vi "State Machine Fundamentals.vi"() -> ()   [LabVIEW 2014]
doc: "Demonstrates the fundamentals of the State Machine design pattern in LabVIEW. A state machine, in its simplest form, is a case structure within a while loop, with a state enum wired to a shift register on the loop to define the execution of different cases (or \"states\") of the case structure on different iterations of the loop."
uses:
  Program Files (x86)/National Instruments/LabVIEW 2014/examples/Design Patterns/State Machine/support/State Machine Fundamentals - State Enum.ctl
panel:
  in  "No":string="No"
  in  "Yes":string="Yes"
  in  "State 3 Text":string="State 3 is executing."
  in  "State 2 Text":string="State 2 is executing. Do you want to execute State 3 next?"
  in  "State 1 Text":string="State 1 is executing."
  in  "Stop":bool
  in  "Run State 2":bool
  in  "Run State 1":bool
  # "Overview: Demonstrates the fundamental concepts of a State Machine design pattern in LabVIEW.\nInstructions:\n1. Run the VI.\n2. Click the Run State 1 button. A dialog pops up displaying text.\n3. Click the Run State 2 button. If you select \"Yes\" in the pop up dialog, State 3 will run after State 2.\n4. Click Stop to stop the VI."
  # "Note: If you are creating a LabVIEW application based on the state machine design pattern, create a Simple State Machine project from the File > Create Project dialog."
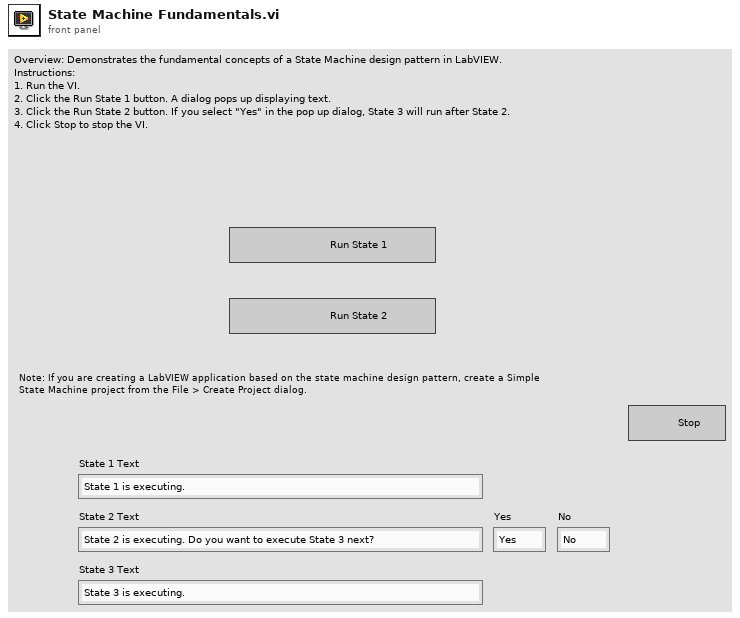
[diagram p1: front panel]
types:
  T1 = typedef "State Machine Fundamentals - State Enum.ctl" = enum16{"Initialize", "Wait for Event", "State 1", "State 2", "State 3", "Stop"}
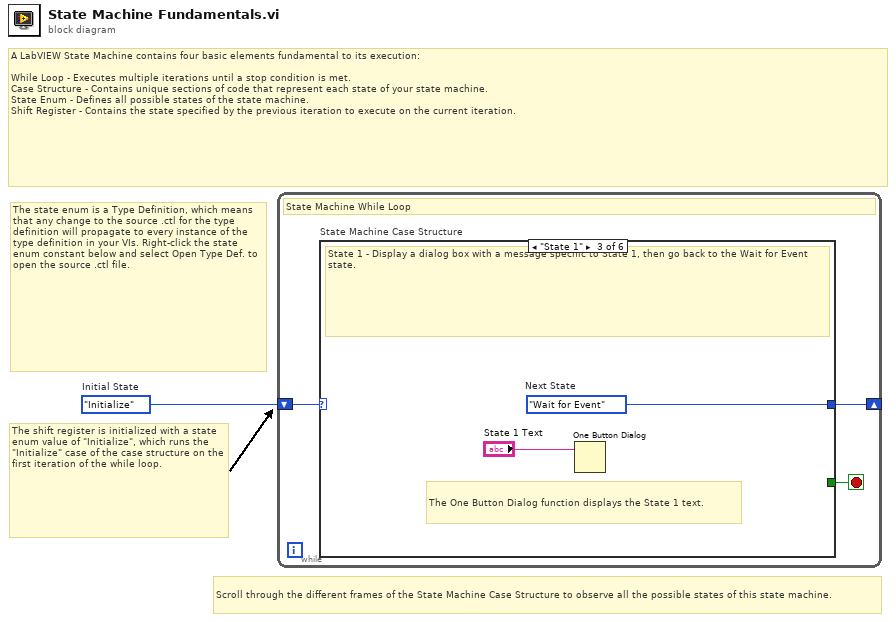
[diagram p0: block diagram]
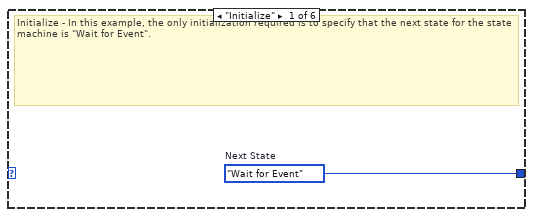
[diagram p2: hidden frame]
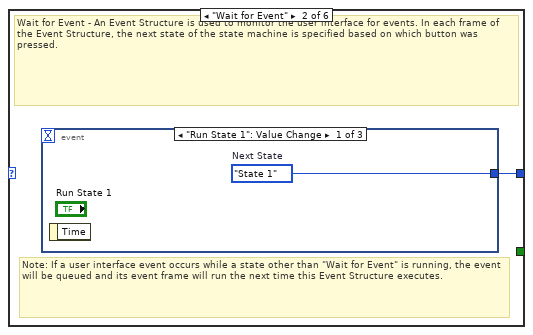
[diagram p3: hidden frame]
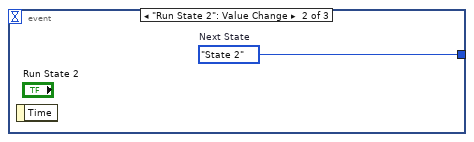
[diagram p4: hidden frame]
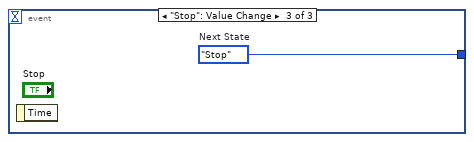
[diagram p5: hidden frame]
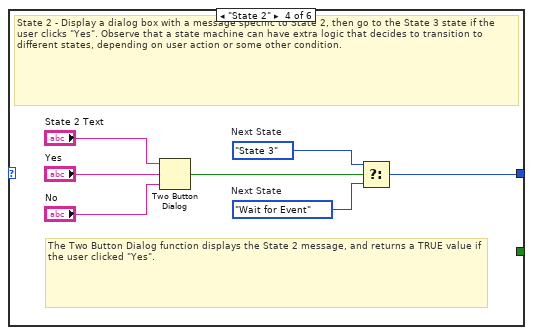
[diagram p6: hidden frame]
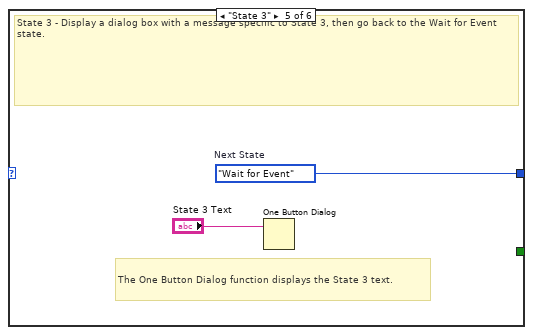
[diagram p7: hidden frame]
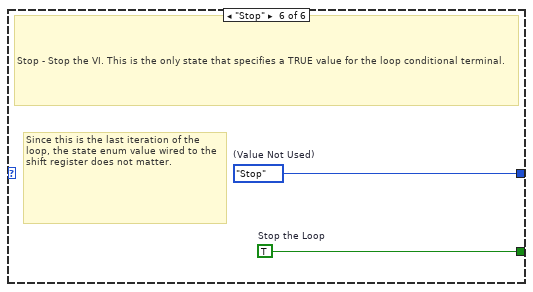
[diagram p8: hidden frame]
diagram:
  w1 = State_Machine_Fundamentals_-_State_Enum."Initialize"  # Initial State
  # "Scroll through the different frames of the State Machine Case Structure to observe all the possible states of this state machine."
  # "The state enum is a Type Definition, which means that any change to the source .ctl for the type definition will propagate to every instance of the type definition in your VIs. Right-click the state enum constant below and select Open Type Def. to open the source .ctl file."
  # "The shift register is initialized with a state enum value of \"Initialize\", which runs the \"Initialize\" case of the case structure on the first iteration of the while loop."
  # "A LabVIEW State Machine contains four basic elements fundamental to its execution:\n\nWhile Loop - Executes multiple iterations until a stop condition is met.\nCase Structure - Contains unique sections of code that represent each state of your state machine.\nState Enum - Defines all possible states of the state machine.\nShift Register - Contains the state specified by the previous iteration to execute on the current iteration."
  n1 = while {
    shift-right: [w3] -> _
    shift-left: w1 -> [w4]
    stop <- w2 stop-if-true
    # "State Machine While Loop"
    n2 = case "State Machine Case Structure" shown="\"State 1\"" w4 {
      tunnel: [w5 w6 w11 w16 w20 w22] -> w3
      tunnel: [_ _ _ _ _ w21] -> w2
      frame "Initialize" {
        w5 = State_Machine_Fundamentals_-_State_Enum."Wait for Event"  # Next State
        # "Initialize - In this example, the only initialization required is to specify that the next state for the state machine is \"Wait for Event\"."
      }
      frame "Wait for Event" {
        # "Note: If a user interface event occurs while a state other than \"Wait for Event\" is running, the event will be queued and its event frame will run the next time this Event Structure executes."
        # "Wait for Event - An Event Structure is used to monitor the user interface for events. In each frame of the Event Structure, the next state of the state machine is specified based on which button was pressed."
        n3 = event shown="[0] \"Run State 1\": Value Change" {
          selector: _ -> [_ _ _]
          dyn-events: _ -> [_ _ _]
          timeout: _ -> [_ _ _]
          tunnel: [w7 w8 w9] -> w6
          event "Run State 1": Value Change {
            w7 = State_Machine_Fundamentals_-_State_Enum."State 1"  # Next State
            n4 = event-data() -> ()  [unwired: 1 in, 1 out]
          }
          event "Run State 2": Value Change {
            w8 = State_Machine_Fundamentals_-_State_Enum."State 2"  # Next State
            n5 = event-data() -> ()  [unwired: 1 in, 1 out]
          }
          event "Stop": Value Change {
            w9 = State_Machine_Fundamentals_-_State_Enum."Stop"  # Next State
            n6 = event-data() -> ()  [unwired: 1 in, 1 out]
          }
        }
      }
      frame "State 1" {
        w11 = State_Machine_Fundamentals_-_State_Enum."Wait for Event"  # Next State
        # "The One Button Dialog function displays the State 1 text."
        # "State 1 - Display a dialog box with a message specific to State 1, then go back to the Wait for Event state."
        n7 = One Button Dialog(message="State 1 Text") -> ()  [unwired: 1 in, 1 out]
      }
      frame "State 2" {
        w15 = State_Machine_Fundamentals_-_State_Enum."Wait for Event"  # Next State
        w17 = State_Machine_Fundamentals_-_State_Enum."State 3"  # Next State
        # "The Two Button Dialog function displays the State 2 message, and returns a TRUE value if the user clicked \"Yes\"."
        # "State 2 - Display a dialog box with a message specific to State 2, then go to the State 3 state if the user clicks \"Yes\". Observe that a state machine can have extra logic that decides to transition to different states, depending on user action or some other condition."
        n8 = Two Button Dialog(message="State 2 Text", 1:"No", 2:"Yes") -> (T button?=w18:bool)
        n9 = Select(t=w17, s=w18, f=w15) -> (s? t:f=w16:T1)
      }
      frame "State 3" {
        w20 = State_Machine_Fundamentals_-_State_Enum."Wait for Event"  # Next State
        # "The One Button Dialog function displays the State 3 text."
        # "State 3 - Display a dialog box with a message specific to State 3, then go back to the Wait for Event state."
        n10 = One Button Dialog(message="State 3 Text") -> ()  [unwired: 1 in, 1 out]
      }
      frame "Stop" {
        w21 = TRUE  # Stop the Loop
        w22 = State_Machine_Fundamentals_-_State_Enum."Stop"  # (Value Not Used)
        # "Since this is the last iteration of the loop, the state enum value wired to the shift register does not matter."
        # "Stop - Stop the VI. This is the only state that specifies a TRUE value for the loop conditional terminal."
      }
    }
  }
